vi "response.To JSON Tree.vi"(8 "error in (no error)":errorcluster, 11 "Response in":refnum<class "Response.lvclass">) -> (0 "error out":errorcluster, 2 "JSON Value out":variant, 3 "Response out":refnum<class "Response.lvclass">)   [LabVIEW 2017, in "Response.lvclass"]
uses:
  Response.lvclass
  Response.lvclass/Response.ctl
  response.Has ID.vi
  response.Has Error.vi
  <vilib>/National Instruments/Variant Data Manipulation/Insert Element at End.vi
  error/error.lvclass
  id/id.lvclass
  result/result.lvclass
  <vilib>/National Instruments/Variant Data Manipulation/Variant Data Manipulation.lvlib
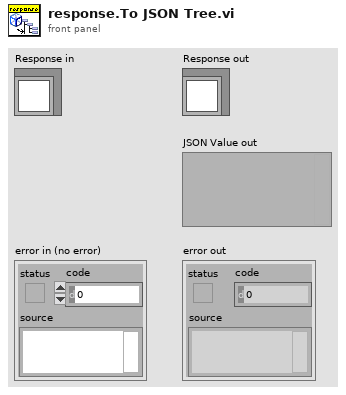
[diagram p1: front panel]
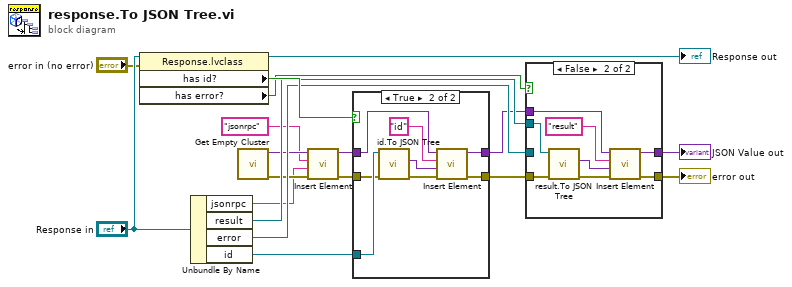
[diagram p0: block diagram]
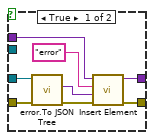
[diagram p2: hidden frame]
diagram:
  n1 = property class="Response.lvclass"(reference="Response in", error in="error in (no error)") -> (reference out=→"Response out":refnum<class "Response.lvclass">, "has id?"=w17:bool, "has error?"=w12:bool)  [unwired: 1 out]
  n2 = Unbundle By Name("Response in") -> ("jsonrpc"=w7:string, "result"=w14:refnum<class "result.lvclass">, "error"=w13:refnum<class "error.lvclass">, "id"=w16:refnum<class "id.lvclass">)
  n3 = call <vilib>:"Get Empty Cluster.vi"() -> ("error out"=w9:errorcluster, "Variant (Cluster) out"=w10:variant)  [unwired: 10 in]
  n4 = call-poly <vilib>:"Insert Element.vi"("error in (no error)"=w9, "element"=w7, "Name"="jsonrpc", "Cluster in"=w10) -> ("error out"=w3:errorcluster, "Cluster out"=w6:variant)  [unwired: 6 in]
  n5 = case shown="True" w17 {
    tunnel: w16 -> [_ w28]
    tunnel: w6 -> [w19 w27]
    tunnel: w3 -> [w20 w24]
    tunnel: [w20 w22] -> w2
    tunnel: [w19 w21] -> w5
    frame False {
    }
    frame True {
      n6 = call "id.To JSON Tree.vi"("error in (no error)"=w24, "id in"=w28) -> ("error out"=w23:errorcluster, "JSON Value out"=w26:variant)  [unwired: 7 in, 1 out]
      n7 = call-poly <vilib>:"Insert Element.vi"("error in (no error)"=w23, "element"=w26, "Name"="id", "Cluster in"=w27) -> ("error out"=w22:errorcluster, "Cluster out"=w21:variant)  [unwired: 6 in]
    }
  }
  n8 = case shown="False" w12 {
    tunnel: w13 -> [w35 _]
    tunnel: w14 -> [_ w40]
    tunnel: w5 -> [w33 w42]
    tunnel: [w32 w41] -> w4
    tunnel: w2 -> [w31 w38]
    tunnel: [w29 w39] -> w1
    frame True {
      n9 = call "error.To JSON Tree.vi"("error in (no error)"=w31, "error in"=w35) -> ("error out"=w30:errorcluster, "JSON Value out"=w34:variant)  [unwired: 7 in, 1 out]
      n10 = call-poly <vilib>:"Insert Element.vi"("error in (no error)"=w30, "element"=w34, "Name"="error", "Cluster in"=w33) -> ("error out"=w29:errorcluster, "Cluster out"=w32:variant)  [unwired: 6 in]
    }
    frame False {
      n11 = call "result.To JSON Tree.vi"("error in (no error)"=w38, "result in"=w40) -> ("error out"=w37:errorcluster, "JSON Value out"=w43:variant)  [unwired: 7 in, 1 out]
      n12 = call-poly <vilib>:"Insert Element.vi"("error in (no error)"=w37, "element"=w43, "Name"="result", "Cluster in"=w42) -> ("error out"=w39:errorcluster, "Cluster out"=w41:variant)  [unwired: 6 in]
    }
  }
  "error out" <- w1
  "JSON Value out" <- w4
